vi "Init Base.vi"(8 "Error In":errorcluster, 10 "Device Name":string, 11 "object in":refnum<class "Instrument.lvclass">) -> (0 "Error Out":errorcluster, 3 "object out":refnum<class "Instrument.lvclass">)   [LabVIEW 2023, in "HAL.lvlib" / "Instrument.lvclass"]
uses:
  Instrument.lvclass
  Instrument.lvclass/Instrument.ctl
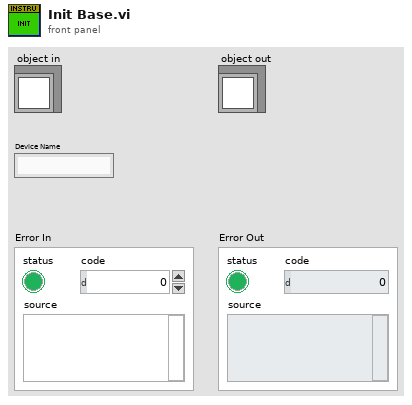
[diagram p1: front panel]
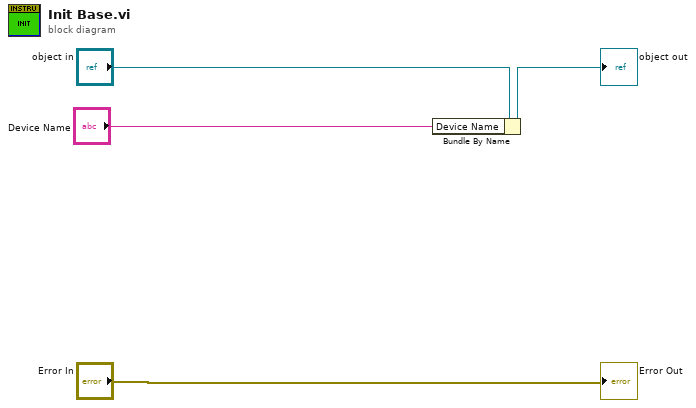
[diagram p0: block diagram]
diagram:
  n1 = Bundle By Name(cluster="object in", "Device Name"="Device Name") -> (→"object out":refnum<class "Instrument.lvclass">)
  "Error Out" <- "Error In"
